vi "hi_cur_data.vi"(9 "length (rest)":i32=5, 10 "regular expression":string, 11 "file path":path=path "C:/luminartech/ManufacturingTools/TS_Automation/Programs/Labview/bring_up/hi_cur/hi_cur_resp.txt") -> (3 "output":i32)   [LabVIEW 2018]
panel:
  out "text":string
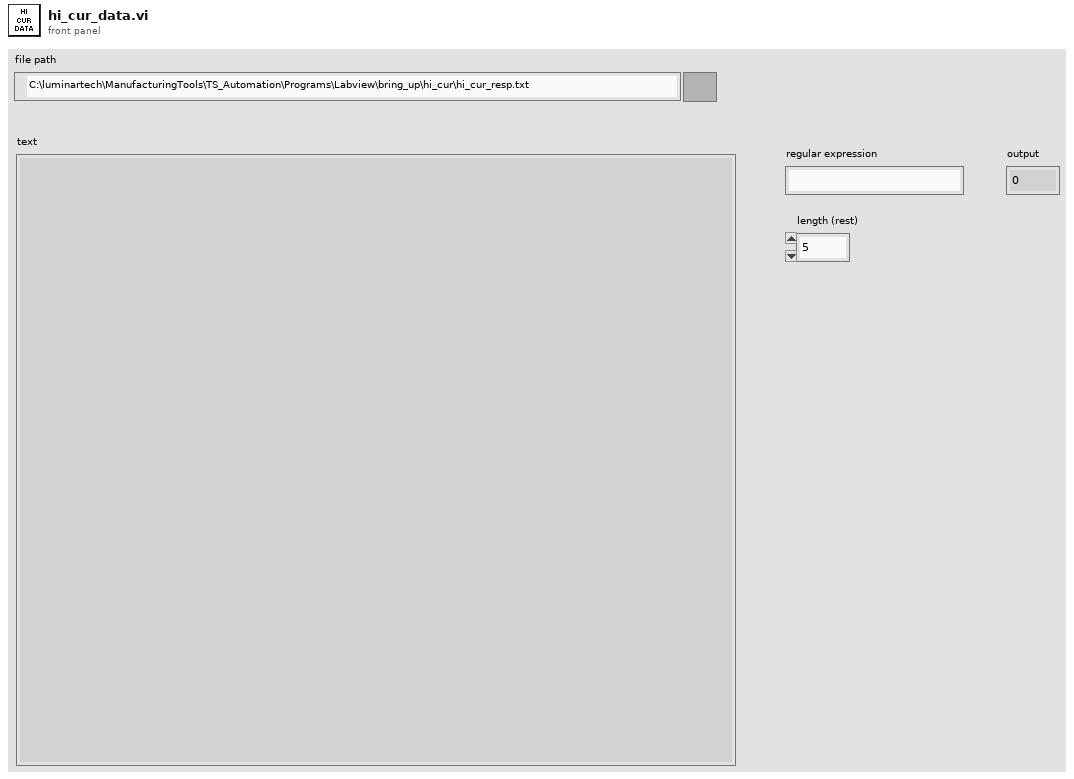
[diagram p1: front panel]
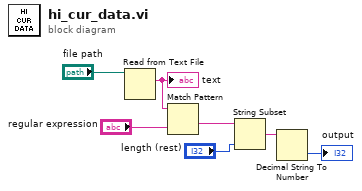
[diagram p0: block diagram]
diagram:
  n1 = Read from Text File(file (use dialog)="file path") -> (text=w6:string)  [unwired: 3 in, 3 out]
  "text" <- w6
  n2 = Match Pattern(string=w6, regular expression="regular expression") -> (after substring=w5:string)  [unwired: 1 in, 3 out]
  n3 = String Subset(string=w5, length (rest)="length (rest)") -> (substring=w4:string)  [unwired: 1 in]
  n4 = Decimal String To Number(string=w4) -> (number=→"output":i32)  [unwired: 2 in, 1 out]
